vi "StopALL.vi"(7 "Write[F]":bool, 11 "StopIN":bool) -> (3 "StopOUT":bool)   [LabVIEW 2014, in "Main.lvlib"]
uses:
  Main.lvlib
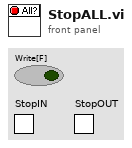
[diagram p1: front panel]
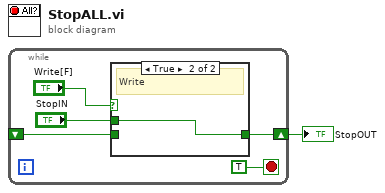
[diagram p0: block diagram]
diagram:
  n1 = while {
    shift-right: [w5] -> w1
    shift-left: _ -> [w4]
    stop <- TRUE stop-if-true
    n2 = case shown="True" "Write[F]" {
      tunnel: [w7 w8] -> w5
      tunnel: w4 -> [w7 _]
      tunnel: "StopIN" -> [_ w8]
      frame False {
        # "Read"
      }
      frame True {
        # "Write"
      }
    }
  }
  "StopOUT" <- w1
